vi "DriveCommandToMotorPower.vi"(6 "Motor Balancing":dbl=1.0, 8 "Drive Command Override":bool, 9 "Drive Command Override (ul) [-1,1]":dbl, 10 "Drive Command (ul) [-1,1]":dbl, 11 "Actual Shifter State":T1(ring)) -> (2 "Motor Power (ul) [-1,1]":dbl)   [LabVIEW 2023]
doc: "This VI linearizes the the drive motor behavior by converting the linear, unitless drive command to the appropriate drive motor power. Handles low and high gear shifter states. The motors shoulds be calibrated with voltage compensation switched ON."
uses:
  GlobalDrivebase.vi
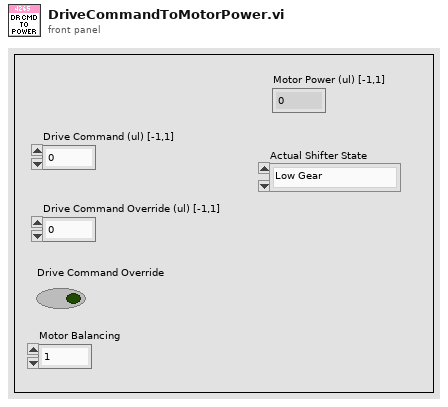
[diagram p1: front panel]
types:
  T1 = enum16{"Low Gear", "High Gear", "Transiting", "Unknown", "Force Low Gear"}
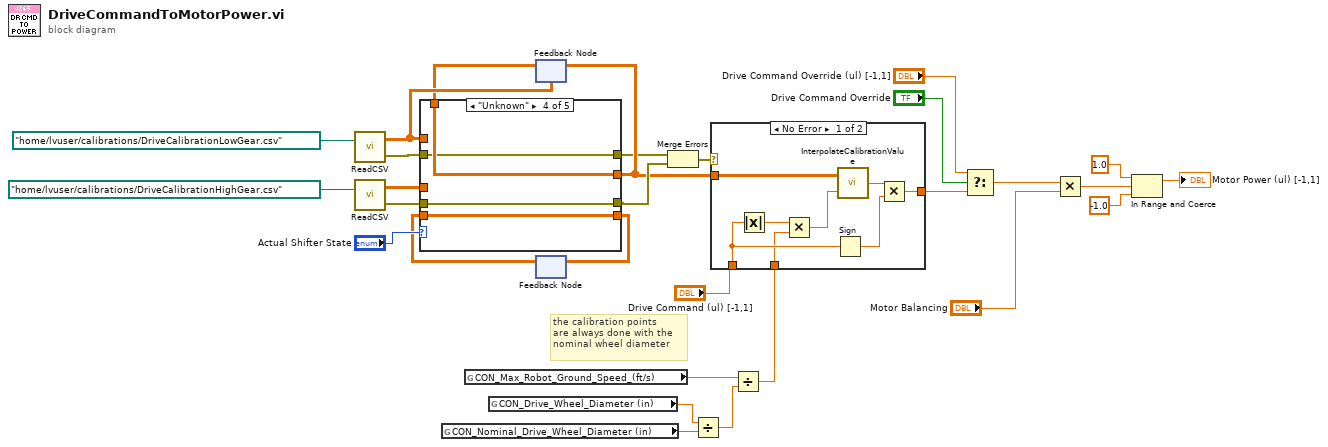
[diagram p0: block diagram]
diagram:
  # "the calibration points\nare always done with the \nnominal wheel diameter"
  n1 = call "ReadCSV.vi"("File Path (.csv)"=path "/home/lvuser/calibrations/DriveCalibrationLowGear.csv" ("path")) -> ("File Open Eror"=w8:errorcluster, "Data (index by row)"=w4:dbl[][])  [unwired: 1 in]
  n2 = call "ReadCSV.vi"("File Path (.csv)"=path "/home/lvuser/calibrations/DriveCalibrationHighGear.csv" ("path")) -> ("File Open Eror"=w6:errorcluster, "Data (index by row)"=w7:dbl[][])  [unwired: 1 in]
  n3 = global read "GlobalDrivebase.vi" "CON_Nominal_Drive_Wheel_Diameter (in)"() -> (w20:dbl)
  n4 = global read "GlobalDrivebase.vi" "CON_Max_Robot_Ground_Speed_(ft/s)"() -> (w18:dbl)
  n5 = global read "GlobalDrivebase.vi" "CON_Drive_Wheel_Diameter (in)"() -> (w19:dbl)
  n6 = feedback #1(w4) -> (w3:dbl[][])
  n7 = feedback #2() -> (w1:dbl[][])  [unwired: 1 in]
  n8 = case shown="\"Unknown\"" "Actual Shifter State" {
    tunnel: w7 -> [w30 w37 _ _ w45]
    tunnel: w4 -> [w33 w34 _ _ w48]
    tunnel: [w33 w37 w38 w44 w48] -> w10
    tunnel: w3 -> [_ _ _ w44 _]
    tunnel: [w32 w36 w40 w43 w47] -> w9
    tunnel: w8 -> [w32 w36 w40 w43 w47]
    tunnel: [w31 w35 w39 w42 w46] -> w11
    tunnel: w6 -> [w31 w35 w39 w42 w46]
    tunnel: [w30 w34 w38 w41 w45] -> w2
    tunnel: w1 -> [_ _ w38 w41 _]
    frame "Low Gear", Default {
    }
    frame "High Gear" {
    }
    frame "Transiting" {
    }
    frame "Unknown" {
    }
    frame "Force Low Gear" {
    }
  }
  n9 = feedback-in #1(w10) -> ()
  n10 = feedback-in #2(w2) -> ()
  n11 = Merge Errors(w9, w11) -> (w27:errorcluster)
  n12 = Divide(x=w19, y=w20) -> (x/y=w17:dbl)
  n13 = Divide(x=w18, y=w17) -> (x/y=w16:dbl)
  n14 = case shown="No Error" w27 {
    tunnel: "Drive Command (ul) [-1,1]" -> [w54 w57]
    tunnel: [w51 w57] -> w26
    tunnel: w10 -> [w50 _]
    tunnel: w16 -> [w49 _]
    frame No Error {
      n15 = Absolute Value(x=w54) -> (abs(x)=w55:dbl)
      n16 = Multiply(x=w55, y=w49) -> (x*y=w56:dbl)
      n17 = Sign(1:w54) -> (0:w52:dbl)
      n18 = call "InterpolateCalibrationValue.vi"("Input"=w56, "Calibration Data"=w50) -> ("Interpolated Output"=w53:dbl)
      n19 = Multiply(x=w53, y=w52) -> (x*y=w51:dbl)
    }
    frame Error {
    }
  }
  n20 = Select(t="Drive Command Override (ul) [-1,1]", s="Drive Command Override", f=w26) -> (s? t:f=w15:dbl)
  n21 = Multiply(x=w15, y="Motor Balancing") -> (x*y=w14:dbl)
  n22 = In Range and Coerce(upper limit=1.0, x=w14, lower limit=-1.0) -> (coerced(x)=→"Motor Power (ul) [-1,1]":dbl)  [unwired: 1 out]
